vi "Dis_Result_Fixture.vi"(4 "Fixture_Data":u16[](array[numeric])) -> (0 "Test_Result_11_20":bool[](array[boolean]), 1 "Test_Result_1_10":bool[](array[boolean]), 2 "Product_Number":u16)   [LabVIEW 2017]
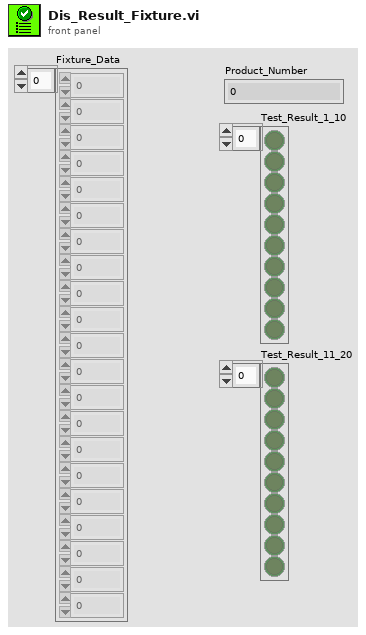
[diagram p1: front panel]
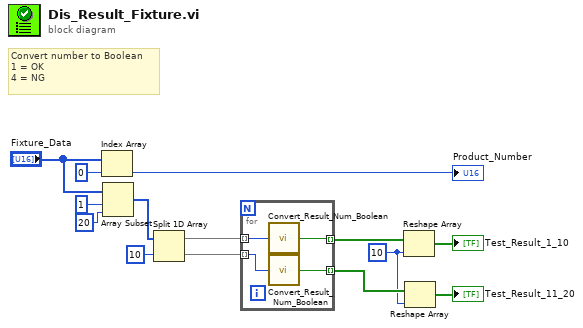
[diagram p0: block diagram]
diagram:
  w5 = 10 ("dimension size")
  # "Convert number to Boolean\n1 = OK\n4 = NG"
  n1 = Index Array(array="Fixture_Data", index=0) -> (element=→"Product_Number":u16)
  n2 = Array Subset(array="Fixture_Data", index=1, length=20) -> (w1:u16[])
  n3 = Split 1D Array(array=w1, index=10) -> (first subarray=w12:u16[], second subarray=w10:u16[])
  n4 = for {
    tunnel: w12 -> [w18] mode=indexing
    tunnel: [w17] -> w9 mode=indexing
    tunnel: w10 -> [w16] mode=indexing
    tunnel: [w15] -> w6 mode=indexing
    n5 = call "Convert_Result_Num_Boolean.vi"("Number_Result"=w18) -> ("Boolean_Result"=w17:bool)  [unwired: 4 in]
    n6 = call "Convert_Result_Num_Boolean.vi"("Number_Result"=w16) -> ("Boolean_Result"=w15:bool)  [unwired: 4 in]
  }
  n7 = Reshape Array(w9, w5) -> (→"Test_Result_1_10":bool[])
  n8 = Reshape Array(w6, w5) -> (→"Test_Result_11_20":bool[])
